vi "Info.vi"(10 "done":dbl, 11 "theta":dbl) -> (0 "theta_min":dbl, 1 "theta_max":dbl, 2 "routine":dbl, 3 "section":i16)   [LabVIEW 2013]
uses:
  <vilib>/Simulation/Implementation/Shared/SIMSCR Execution Mode.ctl
  <vilib>/Simulation/Scripting/Companion Diagram/SimConfigNode/_simSolvers.ctl
  <vilib>/Simulation/Scripting/Companion Diagram/SimConfigNode/SimParams.ctl
  <vilib>/Simulation/Scripting/Companion Diagram/SimConfigNode/SimDog.xnode
  <vilib>/Simulation/Implementation/XNodeFramework/SimXNode/SimX.xnode
  max_min_hold _2(SubVI).vi
  <vilib>/Simulation/Implementation/Shared/NILVSim_FinalizeModel.vi
  <vilib>/Simulation/Implementation/Shared/NILVSim_GetModelError.vi
  <vilib>/Simulation/Implementation/Shared/NILVSim_Initialize.vi
  <vilib>/Simulation/Utility/Implementation/NILVSim Get Time and IsAcceptedStep.vi
  <vilib>/Simulation/Implementation/Shared/NILVSim_Manager.vi
  <vilib>/Simulation/Implementation/Shared/NI_SIM_Implementation.lvlib
  <vilib>/Simulation/Implementation/Shared/NILVSIM_BeginStep.vi
  <vilib>/Simulation/Param Hierarchy/Typedefs/SIMPH Param Control Actions.ctl
  <vilib>/Simulation/Implementation/Shared/NILVSim_ParamChanged.vi
  <vilib>/Utility/error.llb/Clear Errors.vi
  <vilib>/Simulation/Implementation/Shared/SIMSH Read Queue.vi
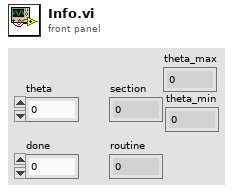
[diagram p1: front panel]
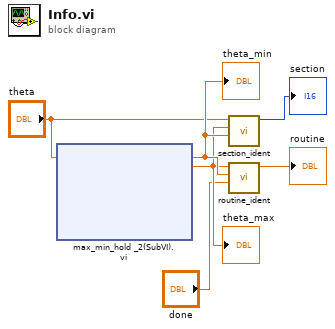
[diagram p0: block diagram]
diagram:
  n1 = xnode "max_min_hold _2(SubVI).vi"("theta"="theta") -> ("theta_min"=w5:dbl, "theta_max"=w4:dbl)  [unwired: 2 in, 10 out]
  "theta_max" <- w4
  "theta_min" <- w5
  n2 = call "section_ident.vi"("theta_min"=w5, "theta_max"=w4, "theta"="theta") -> ("section"=→"section":i16)  [unwired: 8 in]
  n3 = call "routine_ident.vi"("done"="done", "theta_min"=w5, "theta_max"=w4) -> ("routine"=→"routine":dbl)  [unwired: 8 in]
